vi "EF_KaiserFilter.vi"(8 "error in (no error)":errorcluster, 9 "low cutoff freq: fl":dbl=7.0 format="%0.2f", 10 "high cutoff freq: fh":dbl=30.0 format="%0.2f", 11 "Array Of Waveforms in":waveform(dbl)[](array[waveform])) -> (0 "error out":errorcluster, 3 "Filtered Waveforms":waveform(dbl)[](array[waveform]))   [LabVIEW 2016, in "Feature Extraction.lvlib"]
uses:
  <vilib>/Analysis/3filter.llb/Filter Passband Type.ctl
  <vilib>/Analysis/4window.llb/windowTd.ctl
  <vilib>/Analysis/4window.llb/Kaiser-Bessel Window (DBL).vi
  <vilib>/Analysis/2dsp.llb/1D Convolution (DBL).vi
  Feature Extraction.lvlib
  <vilib>/Analysis/NI_AALBase.lvlib
  <vilib>/Analysis/NI_AALPro.lvlib
panel:
  # "This VI is a part of BCI Design library, http://www.ru-bci.org \nCopyright © 2020, Sotnikov Peter, All rights reserved. License: GNU GPLv3"
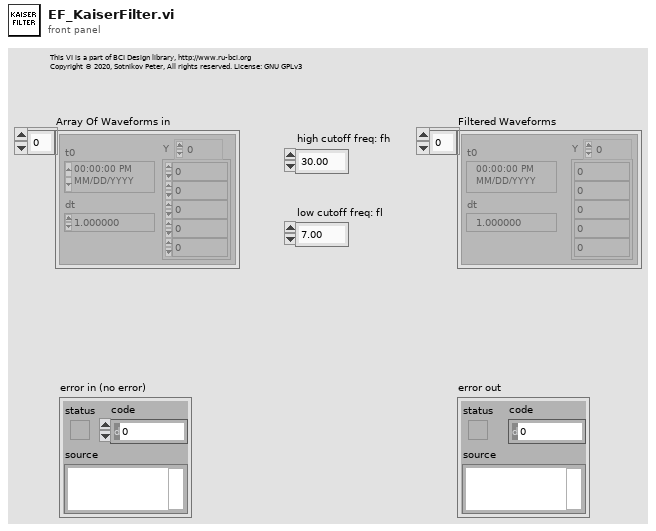
[diagram p1: front panel]
types:
  T1 = typedef "NI_AALPro.lvlib/windowTd.ctl" = u32
  T2 = typedef "NI_AALBase.lvlib/Filter Passband Type.ctl" = enum32{"Lowpass", "Highpass", "Bandpass", "Bandstop"}
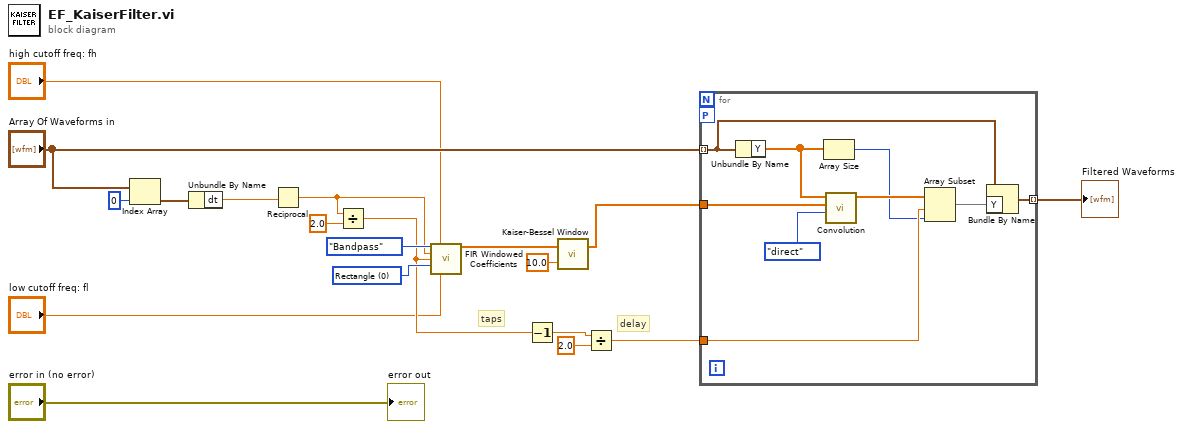
[diagram p0: block diagram]
diagram:
  w13 = T1 0 items=["Rectangle"=0, "Hanning"=1, "Hamming"=2, "Blackman-Harris"=3, "Exact Blackman"=4, "Blackman"=5, "Flat Top"=6, "4 Term B-Harris "=7, "7 Term B-Harris"=8, "Low Sidelobe"=9, "Blackman Nuttall"=11, "Triangle"=30, "Bartlett-Hanning"=31, "Bohman"=32, "Parzen"=33, "Welch"=34, "Kaiser"=60, "Dolph-Chebyshev"=61, "Gaussian"=62] ("window")
  # "delay"
  # "taps"
  n1 = Index Array(array="Array Of Waveforms in", index=0) -> (element=w18:waveform(dbl))
  n2 = Unbundle By Name(w18) -> ("dt"=w16:dbl)
  n3 = Reciprocal(x=w16) -> (1/x=w15:dbl)
  n4 = Divide(x=w15, y=2.0) -> (x/y=w5:dbl)
  n5 = call <vilib>:"FIR Windowed Coefficients.vi"("filter type"=Filter_Passband_Type."Bandpass", "high cutoff freq: fh"="high cutoff freq: fh", "sampling freq: fs"=w15, "taps"=w5, "window"=w13, "low cutoff freq: fl"="low cutoff freq: fl") -> ("FIR Windowed Coefficients"=w12:dbl[])  [unwired: 8 in, 1 out]
  n6 = Decrement(x=w5) -> (x-1=w6:dbl)
  n7 = call-poly <vilib>:"Kaiser-Bessel Window.vi"("beta"=10.0, "X"=w12) -> ("Windowed X"=w9:dbl[])  [unwired: 1 out]
  n8 = Divide(x=w6, y=2.0) -> (x/y=w7:dbl)
  n9 = for {
    tunnel: "Array Of Waveforms in" -> [w21] mode=indexing
    tunnel: w9 -> [w28]
    tunnel: w7 -> [w24]
    tunnel: [w20] -> w3 mode=indexing
    workers-P: _ -> [_]
    n10 = Unbundle By Name(w21) -> ("Y"=w26:dbl[])
    n11 = Array Size(array=w26) -> (size(s)=w23:i32)
    n12 = call-poly <vilib>:"Convolution.vi"("algorithm"=enum32{"direct", "frequency domain"}."direct", "Y"=w28, "X"=w26) -> ("X * Y"=w25:dbl[])  [unwired: 7 in, 1 out]
    n13 = Array Subset(array=w25, index=w24, length=w23) -> (w22:dbl[])
    n14 = Bundle By Name(cluster=w21, "Y"=w22) -> (w20:waveform(dbl))
  }
  "Filtered Waveforms" <- w3
  "error out" <- "error in (no error)"
